vi "VI-Replace Objects in Factory (by name).vi"(0 "LVClassLibrary in":refnum<vi>, 7 "vi path":path, 11 "error in (no error)":errorcluster) -> (4 "reference out":refnum<vi>, 15 "error out":errorcluster)   [LabVIEW 2020]
uses:
  <vilib>/Utility/traverseref.llb/TRef TravTarget.ctl
  <vilib>/Utility/traverseref.llb/VI Scripting - Traverse.lvlib
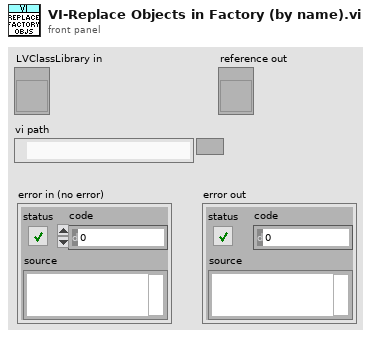
[diagram p1: front panel]
types:
  T1 = typedef "TRef TravTarget.ctl" = enum16{"FP", "BD", "Other"}
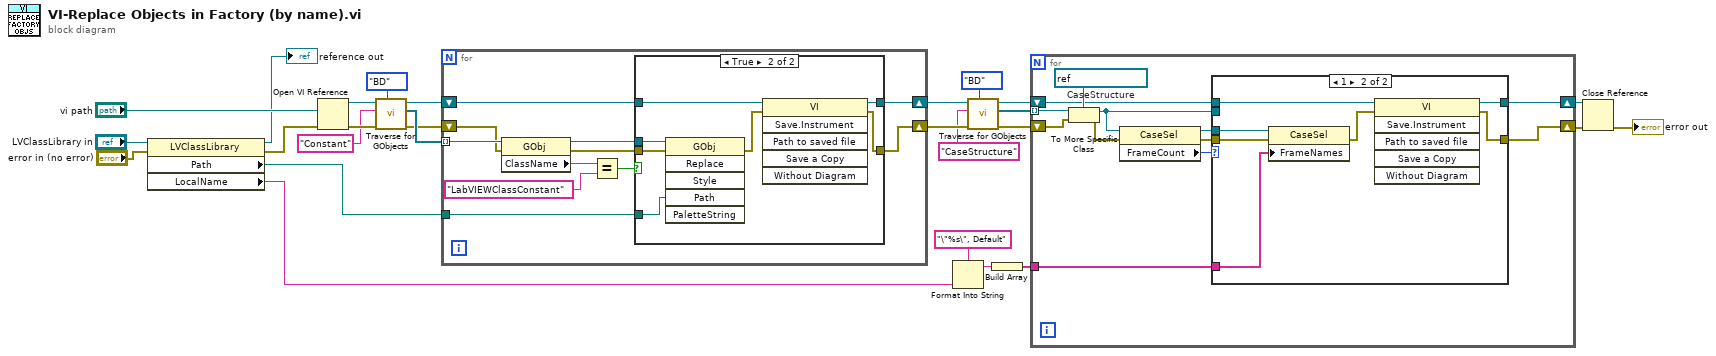
[diagram p0: block diagram]
diagram:
  n1 = property class="LVClassLibrary"(reference="LVClassLibrary in", error in="error in (no error)") -> (reference out=→"reference out":refnum<vi>, error out=w17:errorcluster, "Path"=w16:path, "LocalName"=w4:string)
  n2 = Open VI Reference(vi path="vi path", error in (no error)=w17) -> (vi reference=w27:refnum<vi>, error out=w26:errorcluster)  [unwired: 4 in]
  n3 = call <vilib>:"Traverse for GObjects.vi"("Traverse Target"=TRef_TravTarget."BD", "error in (no error)"=w26, "Class Name"="Constant", "VI Refnum"=w27) -> ("error out"=w22:errorcluster, "References"=w23:refnum<vi>[], "dup VI Refnum"=w20:refnum<vi>)  [unwired: 4 in, 1 out]
  n4 = for {
    tunnel: w23 -> [w38] mode=indexing
    shift-right: [w31] -> w13
    shift-left: w22 -> [w37]
    shift-right: [w29] -> w14
    shift-left: w20 -> [w30]
    tunnel: w16 -> [w28]
    n5 = property class="GObj"(reference=w38, error in=w37) -> (reference out=w34:refnum<vi>, error out=w32:errorcluster, "ClassName"=w36:string)
    n6 = Equal?(x=w36, y="LabVIEWClassConstant") -> (x = y?=w33:bool)
    n7 = case shown="True" w33 {
      tunnel: w34 -> [_ w47]
      tunnel: w32 -> [w40 w46]
      tunnel: [w40 w43] -> w31
      tunnel: w30 -> [w39 w45]
      tunnel: [w39 w42] -> w29
      tunnel: w28 -> [_ w41]
      frame False {
      }
      frame True {
        n8 = invoke class="GObj" method="Replace"(reference=w47, error in=w46, "Path"=w41) -> (error out=w44:errorcluster)  [unwired: 3 in, 5 out]
        n9 = invoke class="VI" method="Save.Instrument"(reference=w45, error in=w44) -> (reference out=w42:refnum<vi>, error out=w43:errorcluster)  [unwired: 4 in, 4 out]
      }
    }
  }
  n10 = Format Into String(format string="\"%s\", Default", w4) -> (resulting string=w3:string)  [unwired: 2 in, 1 out]
  n11 = call <vilib>:"Traverse for GObjects.vi"("Traverse Target"=TRef_TravTarget."BD", "error in (no error)"=w13, "Class Name"="CaseStructure", "VI Refnum"=w14) -> ("error out"=w9:errorcluster, "References"=w7:refnum<vi>[], "dup VI Refnum"=w10:refnum<vi>)  [unwired: 4 in, 1 out]
  n12 = Build Array(w3) -> (w2:string[])
  n13 = for {
    shift-right: [w51] -> w8
    shift-left: w10 -> [w50]
    tunnel: w7 -> [w59] mode=indexing
    shift-right: [w49] -> w6
    shift-left: w9 -> [w57]
    tunnel: w2 -> [w48]
    w58 = refnum<vi> refnum  # CaseStructure
    n14 = To More Specific Class(target class=w58, reference=w59, error in=w57) -> (specific class reference=w52:refnum<vi>, error out=w56:errorcluster)
    n15 = property class="CaseSel"(reference=w52, error in=w56) -> (reference out=w54:refnum<vi>, error out=w53:errorcluster, "FrameCount"=w55:i32)
    n16 = case shown="1" w55 {
      tunnel: w54 -> [_ w68]
      tunnel: w53 -> [w60 w67]
      tunnel: w52 -> [_ _]
      tunnel: [w61 w63] -> w51
      tunnel: w50 -> [w61 w66]
      tunnel: [w60 w64] -> w49
      tunnel: w48 -> [_ w62]
      frame 0, Default {
      }
      frame 1 {
        n17 = property class="CaseSel"(reference=w68, error in=w67, "FrameNames"=w62) -> (error out=w65:errorcluster)  [unwired: 1 out]
        n18 = invoke class="VI" method="Save.Instrument"(reference=w66, error in=w65) -> (reference out=w63:refnum<vi>, error out=w64:errorcluster)  [unwired: 4 in, 4 out]
      }
    }
  }
  n19 = Close Reference(reference=w8, error in (no error)=w6) -> (error out=→"error out":errorcluster)
